vi "Write Protocol type.vi"(8 "error in (no error)":errorcluster, 10 "Protocols":T1, 11 "Protocol in":refnum<class "Protocol.lvclass">) -> (0 "error out":errorcluster, 3 "Protocol out":refnum<class "Protocol.lvclass">)   [LabVIEW 2016, in "Protocol.lvclass"]
uses:
  Protocol.lvclass
  Typedef/Protocol_enum_type.ctl
  Protocol.lvclass/Protocol.ctl
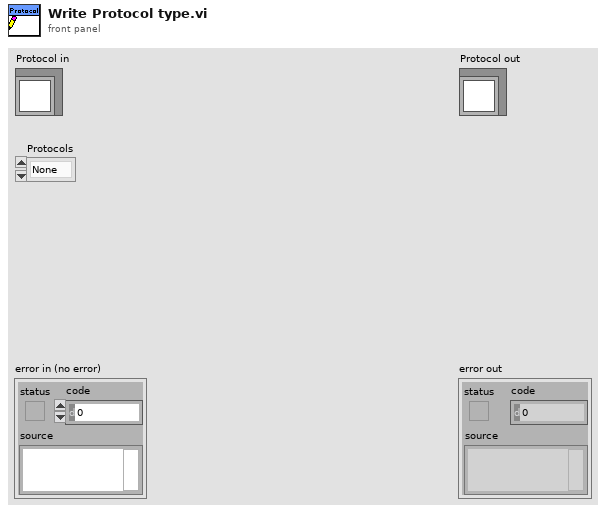
[diagram p1: front panel]
types:
  T1 = typedef "Protocol_enum_type.ctl" = enum16{"None", "MODBUS", "HART", "Fieldbus", "Profibus DP", "Profibus PA", "DeviceNET", "USB"}
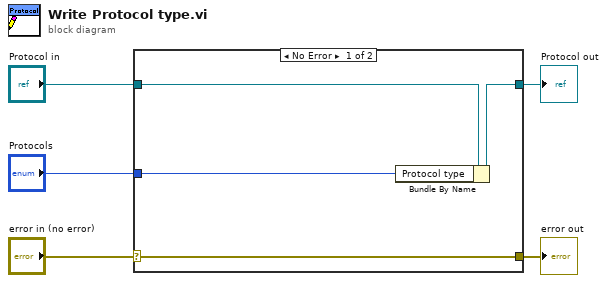
[diagram p0: block diagram]
diagram:
  n1 = case shown="No Error" "error in (no error)" {
    selector: "error in (no error)" -> [w9 w10]
    tunnel: [w9 w10] -> w4
    tunnel: [w7 w11] -> w2
    tunnel: "Protocol in" -> [w8 w11]
    tunnel: "Protocols" -> [w6 _]
    frame No Error {
      n2 = Bundle By Name(cluster=w8, "Protocol type"=w6) -> (w7:refnum<class "Protocol.lvclass">)
    }
    frame Error {
    }
  }
  "error out" <- w4
  "Protocol out" <- w2
